vi "Express Voltage Measurements.vi"(8 "error in":errorcluster, 11 "Input Waveform":waveform(dbl)[](array[waveform])) -> (0 "error out":errorcluster, 1 "Peak to Peak":waveform(dbl)[](graph), 2 "- Peak":waveform(dbl)[](graph), 3 "+ Peak":waveform(dbl)[](graph))   [LabVIEW 2017]
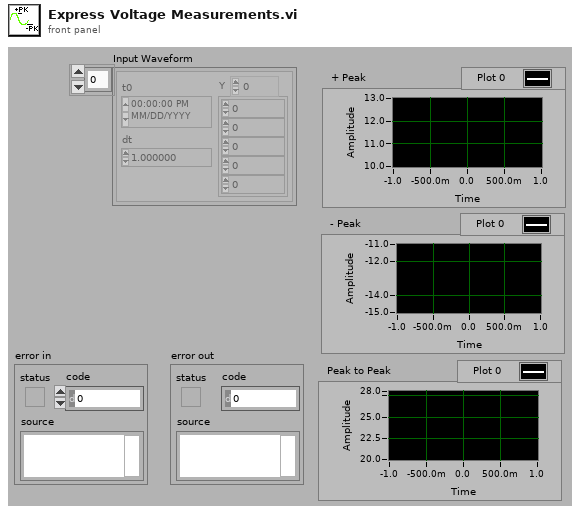
[diagram p1: front panel]
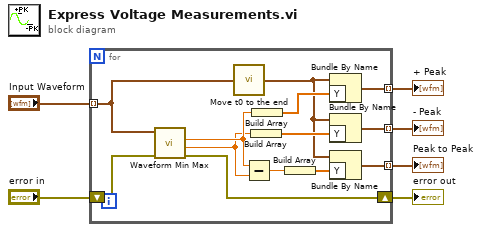
[diagram p0: block diagram]
diagram:
  n1 = for {
    tunnel: "Input Waveform" -> [w8] mode=indexing
    tunnel: [w9] -> w5 mode=indexing
    tunnel: [w17] -> w4 mode=indexing
    tunnel: [w12] -> w3 mode=indexing
    shift-right: [w11] -> w1
    shift-left: "error in" -> [w10]
    n2 = call <vilib>:"Waveform Min Max.vi"("error in (no error)"=w10, "waveform in"=w8) -> ("error out"=w11:errorcluster, "Y min"=w15:dbl, "Y max"=w16:dbl)  [unwired: 4 in, 3 out]
    n3 = call <vilib>:"Move t0 to the end.vi"("waveform in"=w8) -> ("waveform out"=w7:waveform(dbl))
    n4 = Subtract(x=w16, y=w15) -> (x-y=w13:dbl)
    n5 = Build Array(w15) -> (w18:dbl[])
    n6 = Build Array(w16) -> (w19:dbl[])
    n7 = Build Array(w13) -> (w14:dbl[])
    n8 = Bundle By Name(cluster=w7, "Y"=w19) -> (w9:waveform(dbl))
    n9 = Bundle By Name(cluster=w7, "Y"=w18) -> (w17:waveform(dbl))
    n10 = Bundle By Name(cluster=w7, "Y"=w14) -> (w12:waveform(dbl))
  }
  "+ Peak" <- w5
  "- Peak" <- w4
  "Peak to Peak" <- w3
  "error out" <- w1
